vi "Read Props.vi"(8 "error in (no error)":errorcluster, 11 "ButtonControlEditorPanel in":refnum<class "ButtonControlEditorPanel.lvclass">) -> (0 "error out":errorcluster, 2 "Props":T1, 3 "ButtonControlEditorPanel out":refnum<class "ButtonControlEditorPanel.lvclass">)   [LabVIEW 2020, in "VolatusGUIControls.lvlib" / "ButtonControlEditorPanel.lvclass"]
uses:
  ButtonControlEditorPanel.lvclass
  ButtonControlEditorPanel.lvclass/ButtonControlEditorPanel.ctl
  0389b728-1cf1-416b-bf2c-7d7cef5344ff.vi
  <vilib>/JDP Science/JSONtext/JSON text to Variant.vi
  <vilib>/JDP Science/JSONtext/LVClass Serializer/JSONtext LVClass Serializer.lvclass
  VolatusGUIControls.lvlib
  JSON Props.ctl
  VolatusGUIEditorCore/Label Props.ctl
  VolatusGUIEditorCore/VolatusGUIEditorCore.lvlib
  VolatusGUIEditorCore/Position Props.ctl
  VolatusGUIEditorCore/Boolean Color Props.ctl
  VolatusGUIEditorCore/Boolean Text Props.ctl
  Props.ctl
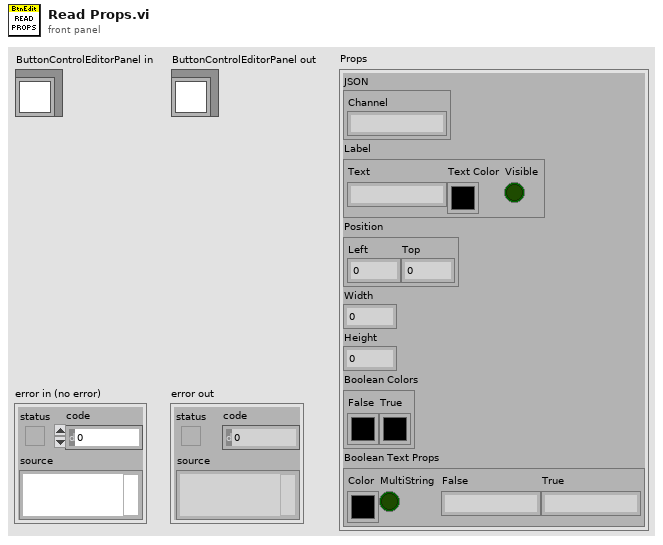
[diagram p1: front panel]
types:
  T1 = typedef "VolatusGUIControls.lvlib/ButtonControlEditorPanel.lvclass/Props.ctl" = cluster{"JSON":T2, "Label":T3, "Position":T4, "Width":u16, "Height":u16, "Boolean Colors":T5, "Boolean Text Props":T6}
  T2 = typedef "VolatusGUIControls.lvlib/ButtonControlEditorPanel.lvclass/JSON Props.ctl" = cluster{"Channel":string}
  T3 = typedef "VolatusGUIEditorCore.lvlib/Label Props.ctl" = cluster{"Text":string, "Text Color":u32, "Visible":bool}
  T4 = typedef "VolatusGUIEditorCore.lvlib/Position Props.ctl" = cluster{"Left":i32, "Top":i32}
  T5 = typedef "VolatusGUIEditorCore.lvlib/Boolean Color Props.ctl" = cluster{"False":u32, "True":u32}
  T6 = typedef "VolatusGUIEditorCore.lvlib/Boolean Text Props.ctl" = cluster{"Color":u32, "MultiString":bool, "False":string, "True":string}
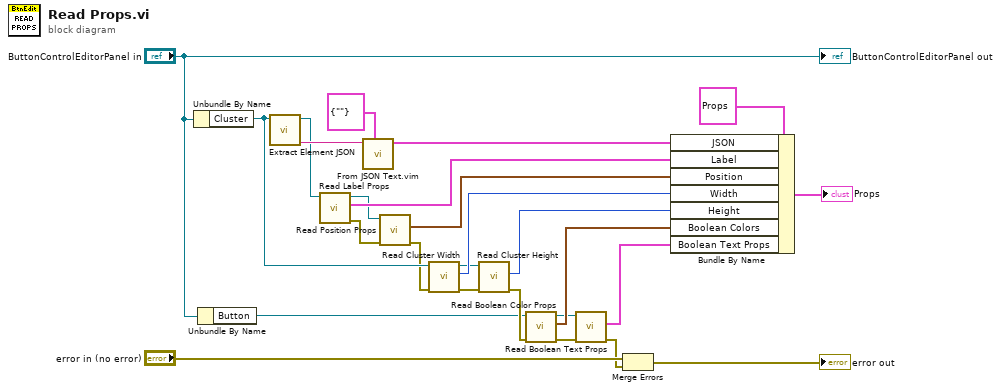
[diagram p0: block diagram]
diagram:
  n1 = Unbundle By Name("ButtonControlEditorPanel in") -> ("Cluster"=w15:refnum<vi>)
  n2 = Unbundle By Name("ButtonControlEditorPanel in") -> ("Button"=w7:refnum<vi>)
  n3 = call "Extract Element JSON.vi"("Ctl Refnum in"=w15) -> ("JSON"=w25:string, "Ctl Refnum"=w19:refnum<vi>)  [unwired: 7 in, 2 out]
  n4 = call "Read Label Props.vi"("Ctl Refnum in"=w19) -> ("error out"=w18:errorcluster, "Label Props"=w20:T3, "Ctl Refnum"=w17:refnum<vi>)  [unwired: 8 in]
  n5 = call "From JSON Text.vim"("Data Type and Default Value"=T2 {"Channel"=""}, "JSON"=w25) -> ("Data out"=w21:T2)  [unwired: 8 in, 1 out]
  n6 = call "Read Position Props.vi"("error in (no error)"=w18, "Ctl Refnum in"=w17) -> ("error out"=w14:errorcluster, "Position Props"=w16:T4)  [unwired: 7 in, 1 out]
  n7 = call "Read Cluster Width.vi"("error in (no error)"=w14, "Cluster in"=w15) -> ("error out"=w11:errorcluster, "Width"=w13:i32, "Cluster"=w12:refnum<vi>)  [unwired: 7 in]
  n8 = call "Read Cluster Height.vi"("error in (no error)"=w11, "Cluster in"=w12) -> ("error out"=w9:errorcluster, "Height"=w10:i32)  [unwired: 7 in, 1 out]
  n9 = call "Read Boolean Color Props.vi"("error in (no error)"=w9, "Control in"=w7) -> ("error out"=w5:errorcluster, "Boolean Colors Props"=w6:T5, "Control"=w4:refnum<vi>)  [unwired: 7 in]
  n10 = call "Read Boolean Text Props.vi"("error in (no error)"=w5, "Control In"=w4) -> ("error out"=w1:errorcluster, "Boolean Text Props"=w3:T6)  [unwired: 7 in, 1 out]
  n11 = Merge Errors("error in (no error)", w1) -> (→"error out":errorcluster)
  n12 = Bundle By Name(cluster=T1 {"JSON"={"Channel"=""}, "Label"={"Text"="", "Text Color"=0, "Visible"=FALSE}, "Position"={"Left"=0, "Top"=0}, "Width"=0, "Height"=0, "Boolean Colors"={"False"=0, "True"=0}, "Boolean Text Props"={"Color"=0, "MultiString"=FALSE, "False"="", "True"=""}} ("Props"), "JSON"=w21, "Label"=w20, "Position"=w16, "Width"=w13, "Height"=w10, "Boolean Colors"=w6, "Boolean Text Props"=w3) -> (→"Props":T1)
  "ButtonControlEditorPanel out" <- "ButtonControlEditorPanel in"
